vi "test events.vi"() -> ()   [LabVIEW 2012]
uses:
  Controls/Wiimote LEDs.ctl
  Class/LV Wiimote Interface.lvclass
panel:
  in  "loop rate":u32=100
  in  "set LEDs?":bool
  out "error out":errorcluster
  in  "Wiimote LEDs In":T1
  in  "stop":bool
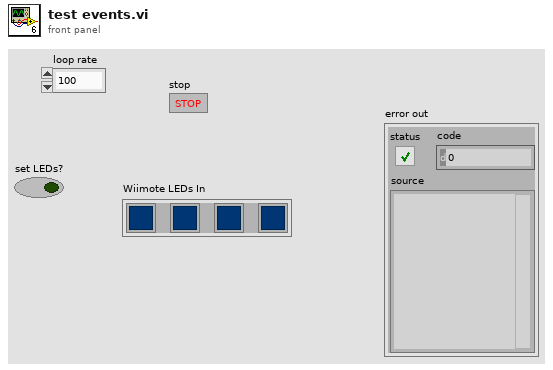
[diagram p1: front panel]
types:
  T1 = typedef "LV Wiimote Interface.lvclass/Wiimote LEDs.ctl" = cluster{"Wiimote LED":bool, "Wiimote LED 2":bool, "Wiimote LED 3":bool, "Wiimote LED 4":bool}
  T2 = typedef "LV Wiimote Interface.ctl" = refnum<class "LV Wiimote Interface.lvclass">
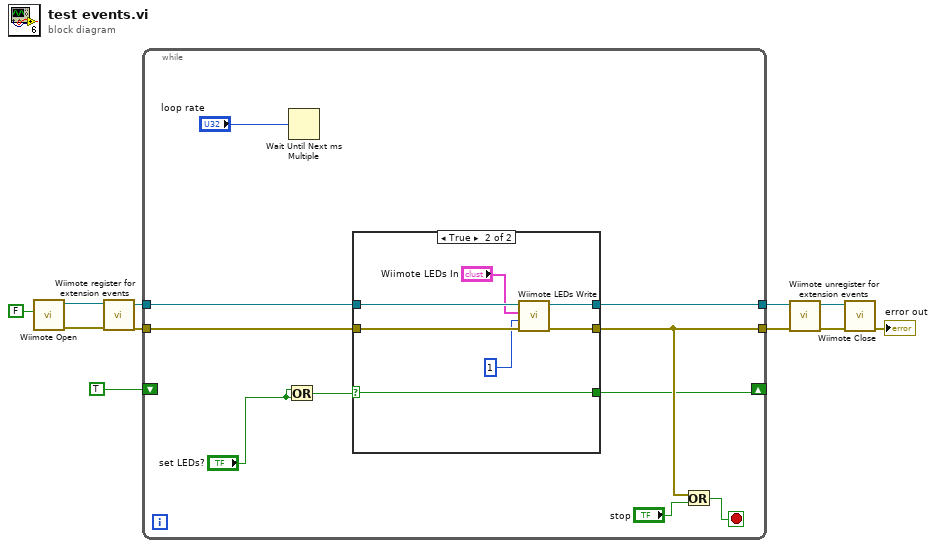
[diagram p0: block diagram]
diagram:
  n1 = call "Wiimote Open.vi"("Connect to all?"=FALSE) -> ("error out"=w9:errorcluster, "LV WiiMote Interface"=w10:T2)  [unwired: 8 in, 1 out]
  n2 = call "Wiimote register for extension events.vi"("error in"=w9, "LV WiiMote Interface In"=w10) -> ("error out"=w7:errorcluster, "LV WiiMote Interface out"=w8:T2)  [unwired: 8 in]
  n3 = while {
    tunnel: w8 -> [w21]
    tunnel: w7 -> [w20]
    tunnel: [w19] -> w4
    tunnel: [w18] -> w2
    shift-right: [w13] -> _
    shift-left: TRUE ("x") -> [_]
    stop <- w16 stop-if-true
    n4 = Or(x="set LEDs?", y="set LEDs?") -> (x .or. y?=w14:bool)
    n5 = Wait Until Next ms Multiple(millisecond multiple="loop rate") -> ()  [unwired: 1 out]
    n6 = case shown="True" w14 {
      selector: w14 -> [w22 w25]
      tunnel: w21 -> [w24 w31]
      tunnel: w20 -> [w23 w30]
      tunnel: [w24 w27] -> w19
      tunnel: [w23 w26] -> w18
      tunnel: [w22 w25] -> w13
      frame False {
      }
      frame True {
        n7 = call "Wiimote LEDs Write.vi"("error in (no error)"=w30, "Wiimote Player #"=1, "Wiimote LEDs In"="Wiimote LEDs In", "LV WiiMote Interface In"=w31) -> ("error out"=w26:errorcluster, "LV WiiMote Interface out"=w27:T2)  [unwired: 5 in, 1 out]
      }
    }
    n8 = Or(x=w18, y="stop") -> (x .or. y?=w16:bool)
  }
  n9 = call "Wiimote unregister for extension events.vi"("error in"=w2, "LV WiiMote Interface In"=w4) -> ("error out"=w1:errorcluster, "LV WiiMote Interface out"=w3:T2)  [unwired: 8 in]
  n10 = call "Wiimote Close.vi"("error in (no error)"=w1, "LV WiiMote Interface"=w3) -> ("error out"=→"error out":errorcluster)  [unwired: 9 in]
